vi "travelError.vi"(8 "error in (no error)":errorcluster, 11 "MoAgSy_AgentBase in":refnum<class "MoAgSy_AgentBase.lvclass">) -> (0 "error out":errorcluster, 3 "MoAgSy_AgentBase out":refnum<class "MoAgSy_AgentBase.lvclass">)   [LabVIEW 2009, in "MoAgSy_Base.lvlib" / "MoAgSy_AgentBase.lvclass"]
uses:
  MoAgSy_AgentBase.lvclass
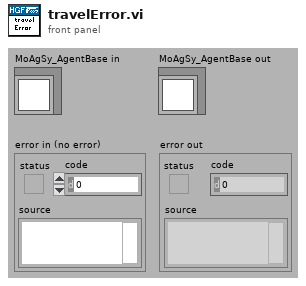
[diagram p1: front panel]
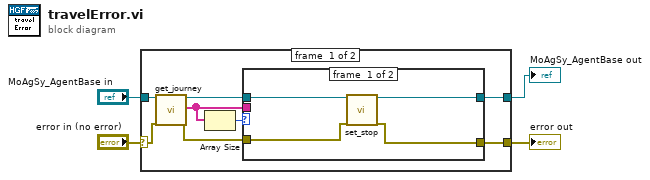
[diagram p0: block diagram]
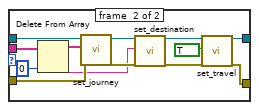
[diagram p2: hidden frame]
diagram:
  n1 = case shown="No Error" "error in (no error)" {
    selector: "error in (no error)" -> [w11 w31]
    tunnel: [w5 w31] -> w3
    tunnel: [w8 w30] -> w1
    tunnel: "MoAgSy_AgentBase in" -> [w12 w30]
    frame #0 {
      n2 = call "get_journey.vi"("HGF_Agent in"=w12, "error in (no error)"=w11) -> ("HGF_Agent out"=w9:refnum<class "MoAgSy_AgentBase.lvclass">, "journey"=w7:string[], "error out"=w6:errorcluster)  [unwired: 15 in]
      n3 = Array Size(array=w7) -> (size(s)=w10:i32)
      n4 = case shown="0, Default" w10 {
        tunnel: w9 -> [w16 w27]
        tunnel: [w15 w22] -> w8
        tunnel: w7 -> [_ w28]
        tunnel: w6 -> [w14 w26]
        tunnel: [w13 w21] -> w5
        frame #0 {
          n5 = call "set_stop.vi"("HGF_Agent.lvclass in"=w16, "error in (no error)"=w14) -> ("HGF_Agent.lvclass out"=w15:refnum<class "MoAgSy_AgentBase.lvclass">, "error out"=w13:errorcluster)  [unwired: 16 in]
        }
        frame #1 {
          n6 = Delete From Array(array=w28, index=0) -> (deleted portion=w18:string, array with subset deleted=w25:string[])  [unwired: 1 in]
          n7 = call "set_journey.vi"("error in (no error)"=w26, "journey"=w25, "MoAgSy_AgentBase in"=w27) -> ("error out"=w19:errorcluster, "MoAgSy_AgentBase out"=w24:refnum<class "MoAgSy_AgentBase.lvclass">)  [unwired: 7 in]
          n8 = call "set_destination.vi"("HGF_Agent in"=w24, "destination"=w18, "error in (no error)"=w19) -> ("HGF_Agent out"=w23:refnum<class "MoAgSy_AgentBase.lvclass">, "error out"=w20:errorcluster)  [unwired: 15 in]
          n9 = call "set_travel.vi"("HGF_Agent in"=w23, "travel?"=TRUE, "error in (no error)"=w20) -> ("HGF_Agent out"=w22:refnum<class "MoAgSy_AgentBase.lvclass">, "error out"=w21:errorcluster)  [unwired: 15 in]
        }
      }
    }
    frame #1 {
    }
  }
  "error out" <- w3
  "MoAgSy_AgentBase out" <- w1
